vi "Chronos TDMS Find All Files in Time Range.vi"(8 "error in (no error)":errorcluster, 9 "path":path, 10 "End Time":timestamp, 11 "Start Time":timestamp) -> (0 "error out":errorcluster, 2 "Time Ranges":T1, 3 "Files":path[](array[path]))   [LabVIEW 2021]
uses:
  typedefs/Chronos cluster Time Ranges.ctl
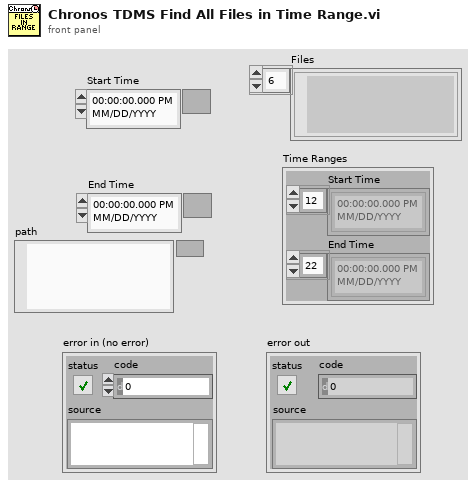
[diagram p1: front panel]
types:
  T1 = typedef "Chronos cluster Time Ranges.ctl" = cluster{"Start Time":timestamp[], "End Time":timestamp[]}
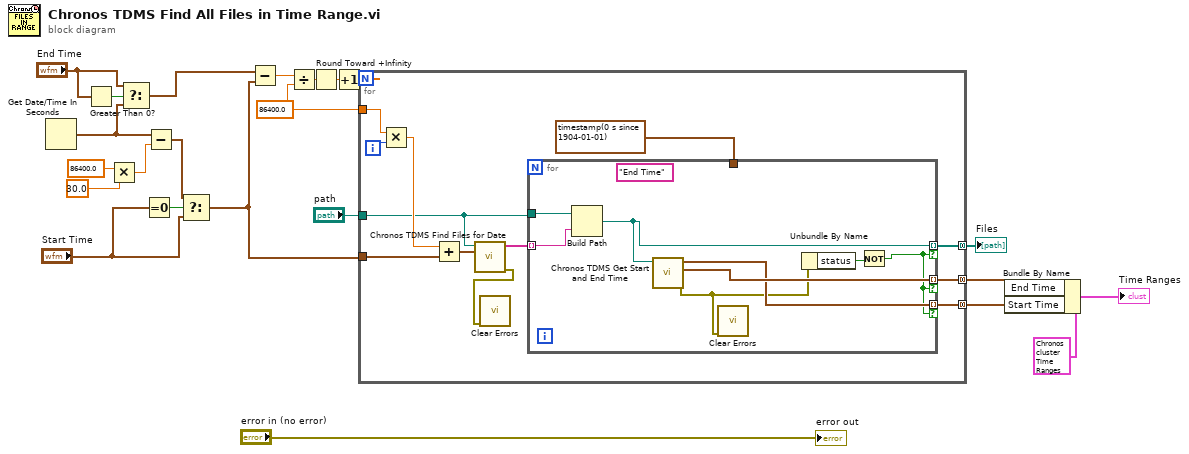
[diagram p0: block diagram]
diagram:
  w20 = 86400.0 ("y")
  n1 = Get Date/Time In Seconds() -> (seconds since 1Jan1904=w8:timestamp)
  n2 = Greater Than 0?(x="End Time") -> (x > 0?=w11:bool)
  n3 = Multiply(x=86400.0 ("y"), y=30.0) -> (x*y=w5:dbl)
  n4 = Select(t="End Time", s=w11, f=w8) -> (s? t:f=w9:timestamp)
  n5 = Equal To 0?(x="Start Time") -> (x = 0?=w12:bool)
  n6 = Subtract(x=w8, y=w5) -> (x-y=w4:timestamp)
  n7 = Select(t=w4, s=w12, f="Start Time") -> (s? t:f=w2:timestamp)
  n8 = Subtract(x=w9, y=w2) -> (x-y=w23:dbl)
  n9 = Divide(x=w23, y=w20) -> (x/y=w22:dbl)
  n10 = Round Toward +Infinity(x=w22) -> (ceil(x): smallest int >= x=w21:dbl)
  n11 = Increment(x=w21) -> (x+1=w13:dbl)
  n12 = for {
    N: w13 -> [_]
    tunnel: w20 -> [w33]
    tunnel: w2 -> [w30]
    tunnel: [w28] -> w16 mode=concatenating
    tunnel: [w27] -> w18 mode=concatenating
    tunnel: [w26] -> w17 mode=concatenating
    tunnel: "path" -> [w25]
    i -> [w32]
    n13 = Multiply(x=w33, y=w32) -> (x*y=w31:dbl)
    n14 = Add(x=w31, y=w30) -> (x+y=w29:timestamp)
    n15 = call "Chronos TDMS Find Files for Date.vi"("time stamp"=w29, "path"=w25) -> ("error out"=w24:errorcluster, "files"=w35:string[])  [unwired: 7 in, 1 out]
    n16 = call <vilib>:"Clear Errors.vi"("error in (no error)"=w24) -> ()  [unwired: 5 in, 2 out]
    n17 = for {
      tunnel: w25 -> [w43]
      tunnel: w35 -> [w42] mode=indexing
      tunnel: timestamp(0 s since 1904-01-01) -> [_]
      tunnel: [w40] -> w28 mode=indexing if=w36
      tunnel: [w39] -> w27 mode=indexing if=w36
      tunnel: [w41] -> w26 mode=indexing if=w36
      (unwired) "End Time" ("group name")
      n18 = Build Path(base path=w43, name or relative path=w42) -> (appended path=w39:path)
      n19 = call "Chronos TDMS Get Start and End Time.vi"("file path"=w39) -> ("error out"=w38:errorcluster, "end time"=w41:timestamp, "Start time"=w40:timestamp)  [unwired: 8 in]
      n20 = call <vilib>:"Clear Errors.vi"("error in (no error)"=w38) -> ()  [unwired: 5 in, 2 out]
      n21 = Unbundle By Name(w38) -> ("status"=w37:bool)
      n22 = Not(x=w37) -> (.not. x?=w36:bool)
    }
  }
  "Files" <- w18
  n23 = Bundle By Name(cluster=T1 {"Start Time"=[timestamp(3663856443.7469993 s since 1904-01-01), timestamp(0 s since 1904-01-01)], "End Time"=[timestamp(3663856162.166964 s since 1904-01-01), timestamp(3663856456.345259 s since 1904-01-01)]} ("Time Ranges"), "End Time"=w17, "Start Time"=w16) -> (→"Time Ranges":T1)
  "error out" <- "error in (no error)"
